vi "readSVs.vi"(8 "error in (no error)":errorcluster, 11 "ComponentData in":refnum<class "ComponentData.lvclass">) -> (0 "error out":errorcluster, 3 "ComponentData out":refnum<class "ComponentData.lvclass">)   [LabVIEW 2013, in "ComponentData.lvlib" / "ComponentData.lvclass"]
uses:
  <userlib>/Common/Component/common_application/RT/ComponentData/ComponentData/ComponentData.lvclass
  <userlib>/Common/Component/common_application/RT/ComponentData/ComponentData/ComponentData.lvclass/ComponentData.ctl
  <userlib>/Common/Component/common_application/RT/ComponentData/ApplicationHandler/ApplicationHandler.lvclass
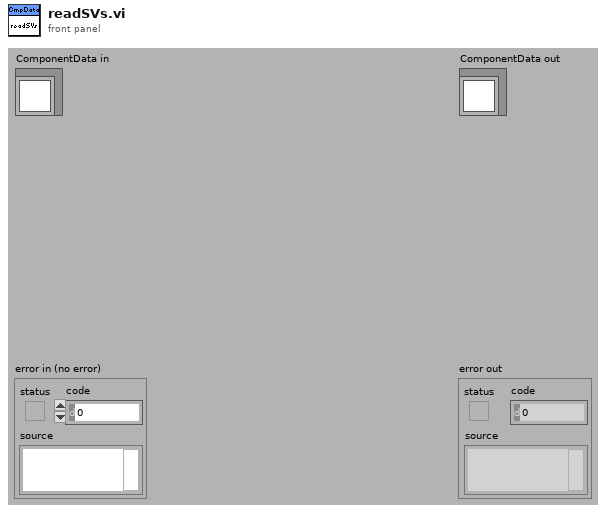
[diagram p1: front panel]
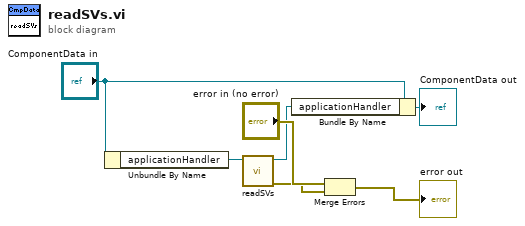
[diagram p0: block diagram]
diagram:
  n1 = Unbundle By Name("ComponentData in") -> ("applicationHandler"=w7:refnum<class "ApplicationHandler.lvclass">)
  n2 = call <userlib>:"readSVs.vi"("ApplicationHandler in"=w7) -> ("error out"=w5:errorcluster, "ApplicationHandler out"=w2:refnum<class "ApplicationHandler.lvclass">)  [unwired: 9 in]
  n3 = Bundle By Name(cluster="ComponentData in", "applicationHandler"=w2) -> (→"ComponentData out":refnum<class "ComponentData.lvclass">)
  n4 = Merge Errors("error in (no error)", w5) -> (→"error out":errorcluster)
